vi "20TILM_Split_Cluster.vi"(0 "20TILM":T3) -> (1 "20TILM Status":T2, 2 "20T Control":T1)   [LabVIEW 2019]
uses:
  Gustav/20TILM_Cluster.ctl
  Gustav/20TILM_Status.ctl
  Gustav/20TILM_Control.ctl
panel:
  # "Levelmeter"
  # "Helium (%)"
  # "Levelmeter"
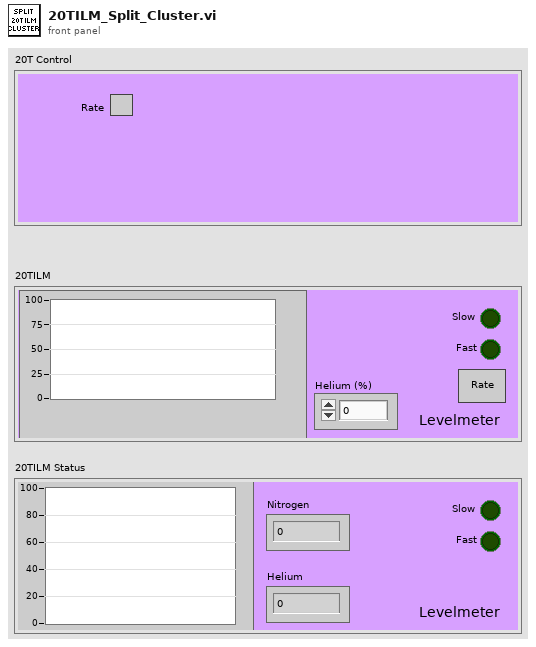
[diagram p1: front panel]
types:
  T1 = typedef "20TILM_Control.ctl" = cluster{"Rate":bool}
  T2 = typedef "20TILM_Status.ctl" = cluster{"Helium":dbl, "Nitrogen":dbl, "Slow":bool, "Fast":bool, "Plot":cluster{"X":dbl, "Y":dbl}[]}
  T3 = typedef "20TILM_Cluster.ctl" = cluster{"Helium":dbl, "Nitrogen":dbl, "Slow":bool, "Fast":bool, "Plot":cluster{"X":dbl, "Y":dbl}[], "Rate":bool}
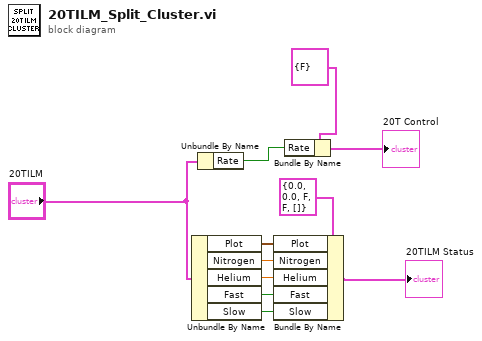
[diagram p0: block diagram]
diagram:
  n1 = Unbundle By Name("20TILM") -> ("Plot"=w11:cluster{"X":dbl, "Y":dbl}[], "Nitrogen"=w10:dbl, "Helium"=w9:dbl, "Fast"=w8:bool, "Slow"=w7:bool)
  n2 = Unbundle By Name("20TILM") -> ("Rate"=w6:bool)
  n3 = Bundle By Name(cluster=T2 {"Helium"=0.0, "Nitrogen"=0.0, "Slow"=FALSE, "Fast"=FALSE, "Plot"=[]} ("20TILM Status"), "Plot"=w11, "Nitrogen"=w10, "Helium"=w9, "Fast"=w8, "Slow"=w7) -> (→"20TILM Status":T2)
  n4 = Bundle By Name(cluster=T1 {"Rate"=FALSE} ("SR830-2 2"), "Rate"=w6) -> (→"20T Control":T1)
